vi "Error Handler Queue.vi"(8 "error in (no error)":errorcluster, 11 "LogRotate in":refnum<class "LogRotate.lvclass">) -> (0 "error out":errorcluster)   [LabVIEW 2021, in "Error_Manager.lvlib" / "LogRotate.lvclass"]
uses:
  LogRotate.lvclass
  LogRotate.lvclass/LogRotate.ctl
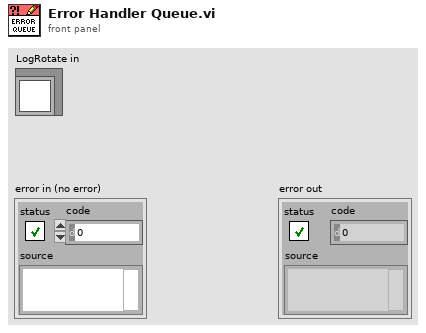
[diagram p1: front panel]
types:
  T1 = typedef "Error_Manager.lvlib/LogRotate.lvclass/LogData.ctl" = cluster{"error constant":errorcluster, "replacements":string[], "Time Stamp":timestamp}
  T2 = enum32{"Bad", "Idle", "Run top level", "Running"}
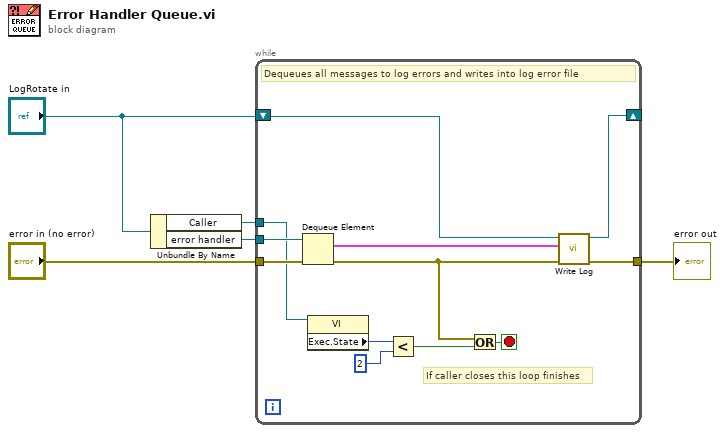
[diagram p0: block diagram]
diagram:
  n1 = Unbundle By Name("LogRotate in") -> ("Caller"=w1:refnum<vi>, "error handler"=w3:refnum<queue>)
  n2 = while {
    tunnel: w3 -> [w16]
    tunnel: w1 -> [w10]
    shift-right: [w6] -> _
    shift-left: "LogRotate in" -> [w14]
    tunnel: "error in (no error)" -> [w17]
    tunnel: [w15] -> w4
    stop <- w11 stop-if-true
    # "If caller closes this loop finishes"
    # "Dequeues all messages to log errors and writes into log error file"
    n3 = Dequeue Element(queue=w16, error in (no error)=w17) -> (element=w13:T1, error out=w12:errorcluster)  [unwired: 1 in, 2 out]
    n4 = property class="VI"(reference=w10) -> ("Exec.State"=w9:T2)  [unwired: 1 in, 2 out]
    n5 = Less?(x=w9, y=2) -> (x < y?=w7:bool)
    n6 = Or(x=w12, y=w7) -> (x .or. y?=w11:bool)
    n7 = call "Write Log.vi"("error in (no error)"=w12, "LogData"=w13, "LogRotate in"=w14) -> ("error out"=w15:errorcluster, "LogRotate out"=w6:refnum<class "LogRotate.lvclass">)  [unwired: 7 in]
  }
  "error out" <- w4
